vi "Wind Farm #2.vi"(8 "error in (no error)":errorcluster) -> (0 "error out":errorcluster)   [LabVIEW 2011]
doc: "This is one of 4 potential implementations for the Wind Farm Requirements. Specifically note how the wind turbine information is displayed. Also note how the main VI communicates back and forth to the wind turbine. What does that pipeline look like? Finally note the mechanism for stopping the wind turbine.\n\nAAL 9/09"
uses:
  Controls/File Type.ctl
  X Listbox Solution/X Listbox-Solution.xctl
  Shared/QDMH Poly VIs/QDMH POLY Enqueue String.vi
  Shared/QDMH Poly VIs/QDMH POLY Enqueue Cluster.vi
panel:
  in  "Wind Turbine Selection":string(xcontrol)
  in  "File Type":T1 caption="File Type (Read When Turbine is Added)"
  in  "Set Wind Speed":bool
  in  "Wind Speed":dbl=15.0
  in  "Queue Name":string
  in  "Add Wind Turbine":bool
  out "Message Display":string
  in  "Exit":bool
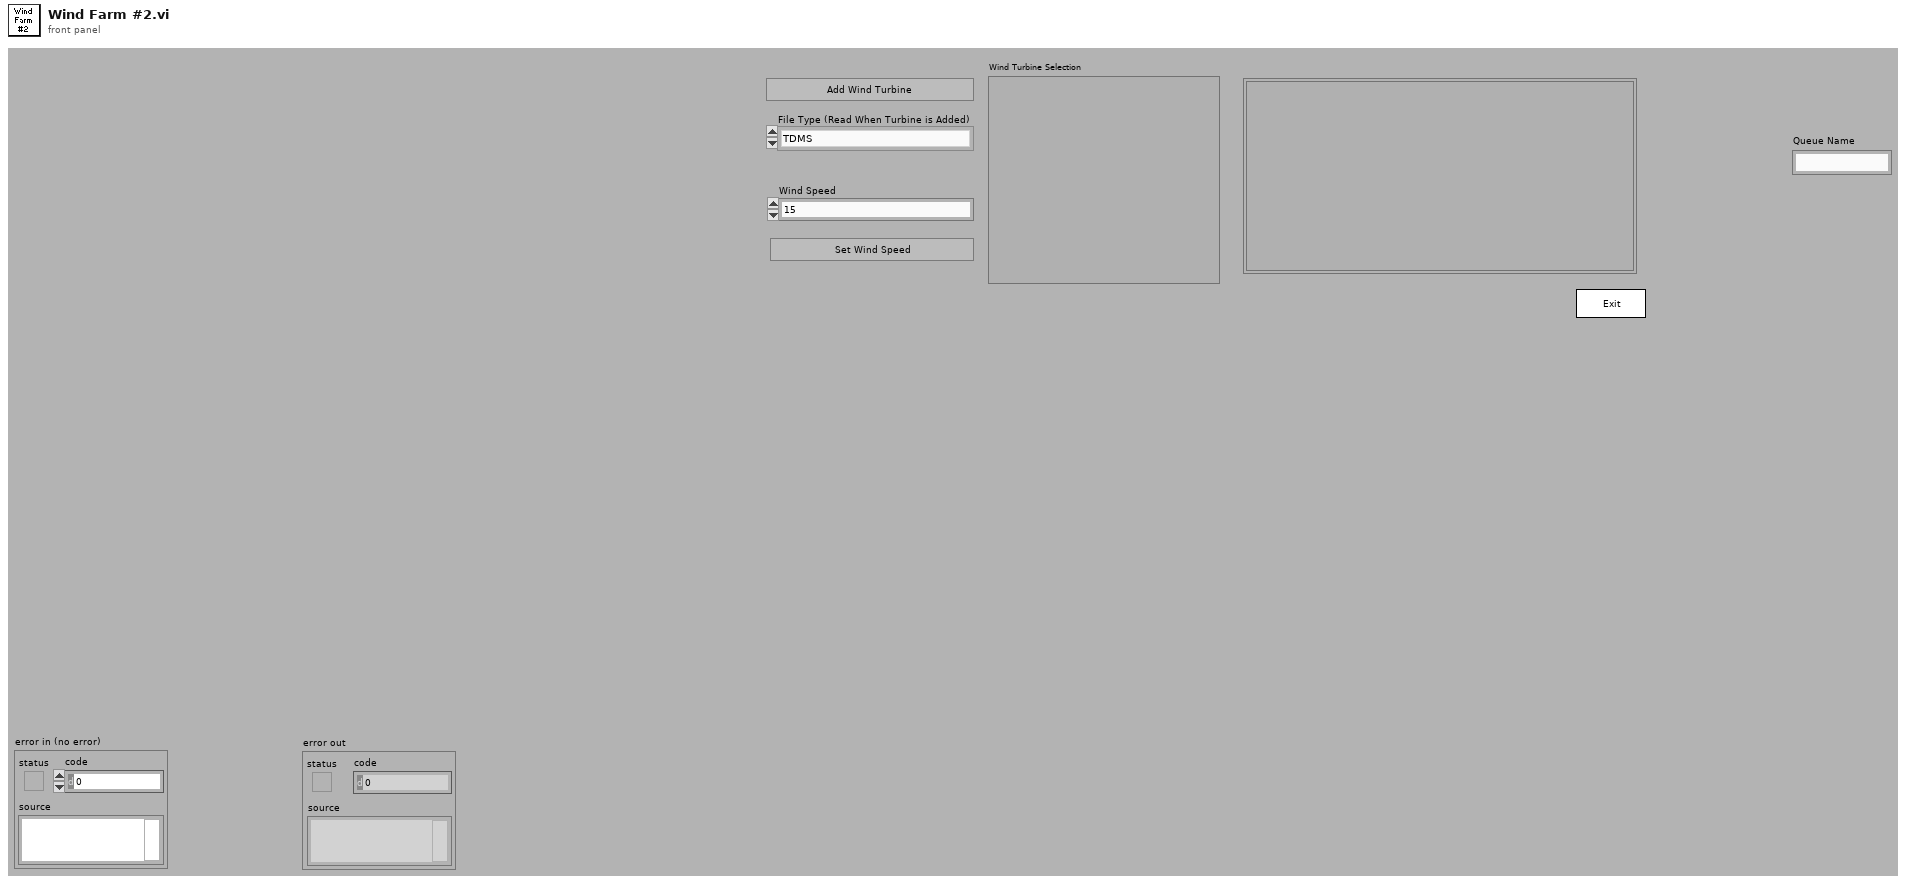
[diagram p1: front panel]
types:
  T1 = typedef "File Type.ctl" = enum16{"TDMS", "TXT"}
  T2 = cluster{"Operator Name":string, "Current VI's  Path":path, "Main Directory":path, "Y Data":dbl[], "Ini Path":path, "Model":string, "VITs Directory":path, "VIT References":refnum<vi>[], "VIT Current":refnum<vi>, "Wind Speed":dbl, "Selected Turbine":string, "Names":string[]}
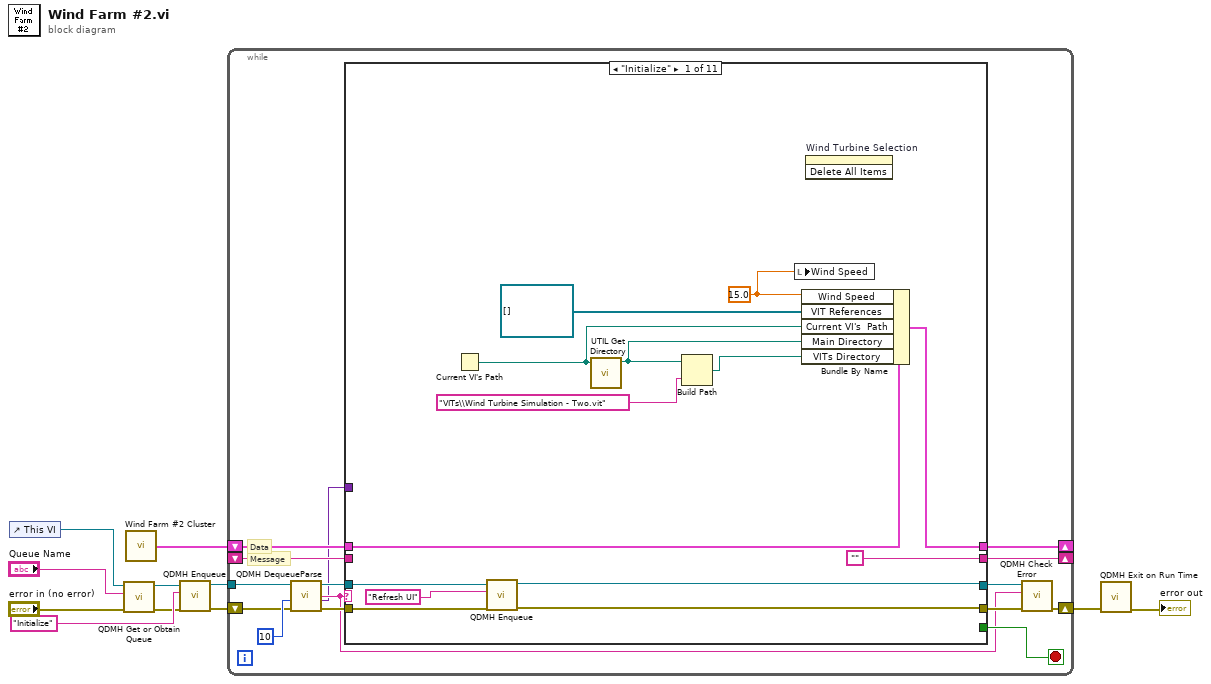
[diagram p0: block diagram]
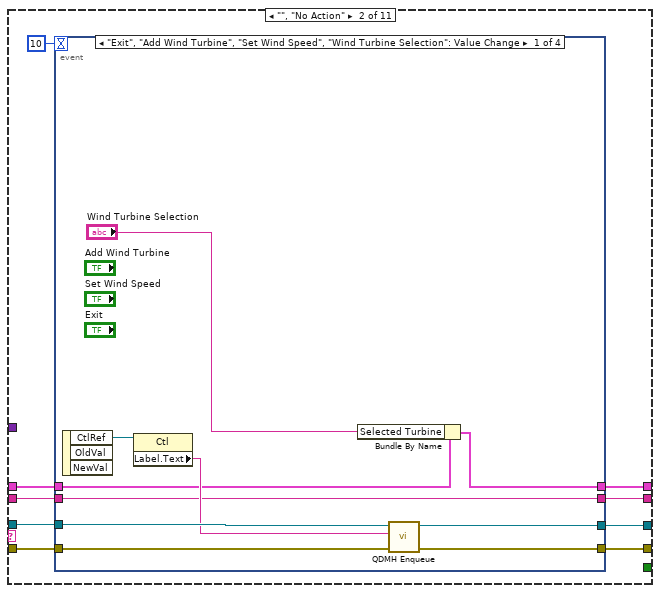
[diagram p2: hidden frame]
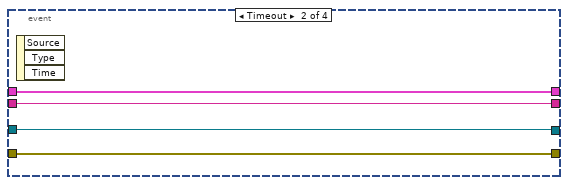
[diagram p3: hidden frame]
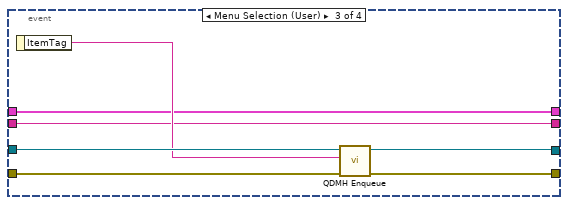
[diagram p4: hidden frame]
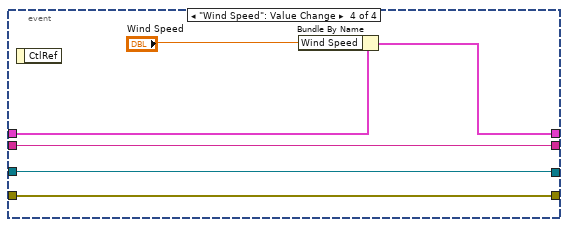
[diagram p5: hidden frame]
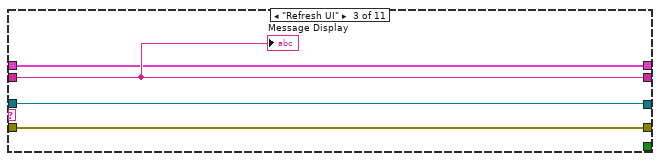
[diagram p6: hidden frame]
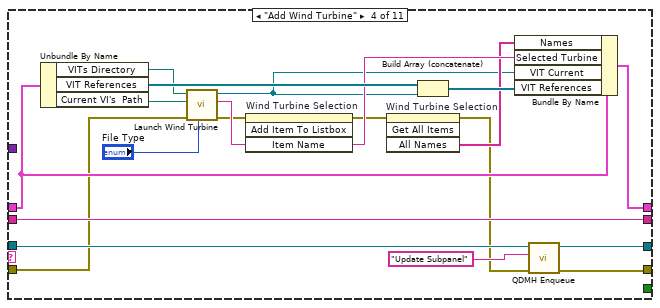
[diagram p7: hidden frame]
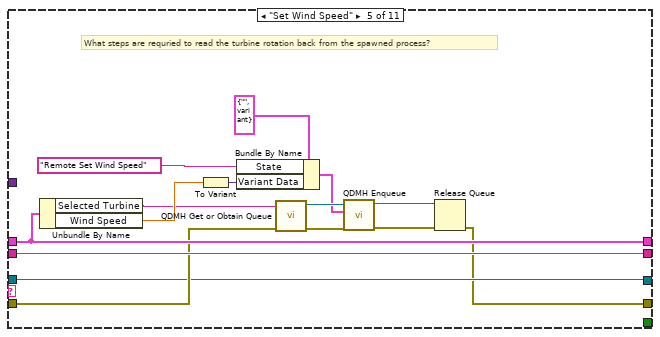
[diagram p8: hidden frame]
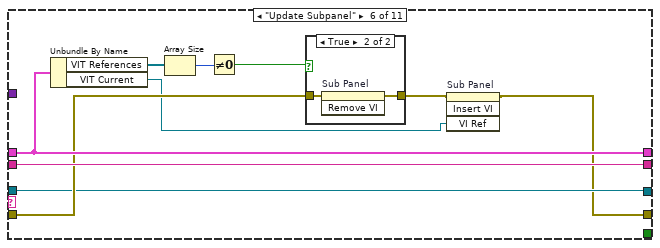
[diagram p9: hidden frame]
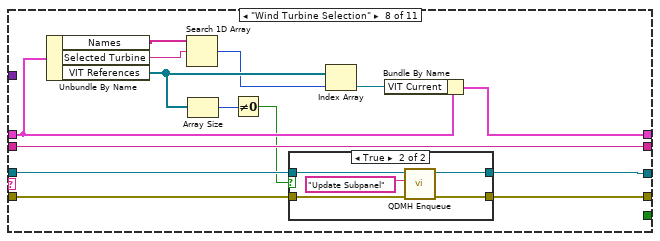
[diagram p12: hidden frame]
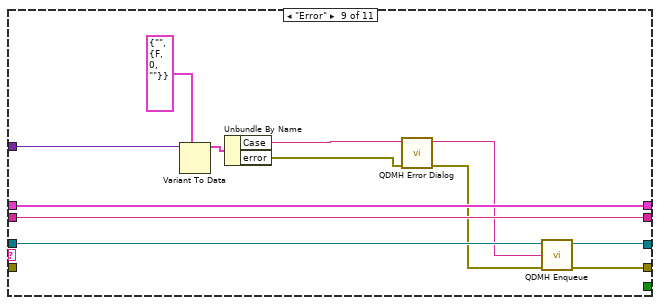
[diagram p14: hidden frame]
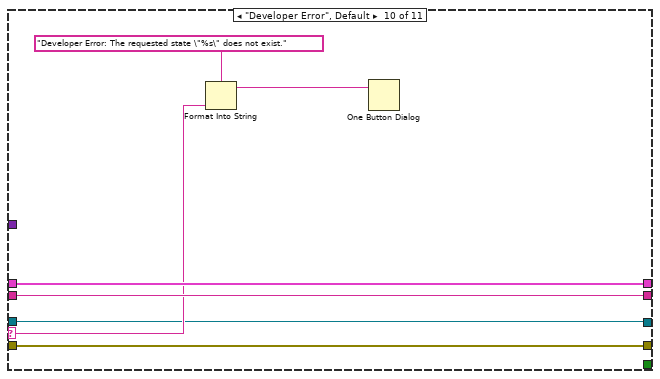
[diagram p15: hidden frame]
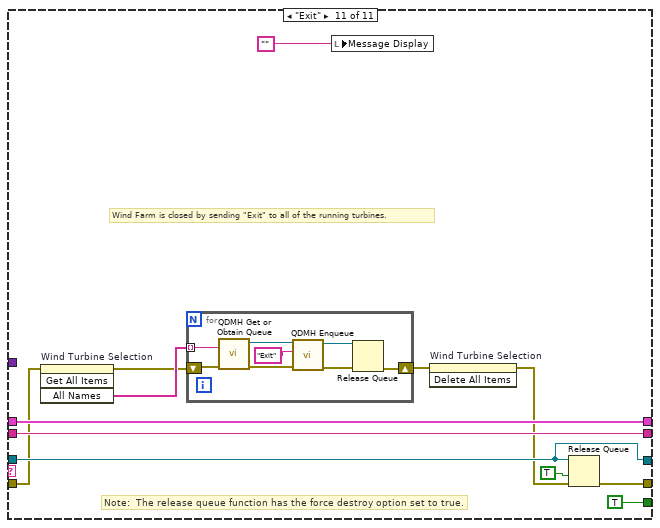
[diagram p16: hidden frame]
diagram:
  n1 = control-ref of="This VI"() -> (w1:refnum<vi>)
  n2 = call "QDMH Get or Obtain Queue.vi"("error in (no error)"="error in (no error)", "Queue Name"="Queue Name", "VI Refnum"=w1) -> ("error out"=w7:errorcluster, "queue out"=w10:refnum<queue>)  [unwired: 7 out]
  n3 = call "Wind Farm #2 Cluster.vi"() -> ("Cluster"=w3:T2)
  n4 = call-poly "QDMH Enqueue.vi"("error in (no error)"=w7, "State"="Initialize" ("element"), "queue"=w10) -> ("error out"=w8:errorcluster, "queue out"=w11:refnum<queue>)  [unwired: 7 out]
  n5 = while {
    tunnel: w11 -> [w21]
    shift-left: w3 -> [w22]
    shift-right: [w23] -> _
    shift-left: _ -> [w24]
    shift-right: [w25] -> _
    shift-right: [w15] -> w5
    shift-left: w8 -> [w17]
    stop <- w26 stop-if-true
    # "Data"
    # "Message"
    n6 = call "QDMH DequeueParse.vi"("error in (no error)"=w17, "Timeout"=10 ("ms timeout (-1)"), "queue"=w21) -> ("error out"=w18:errorcluster, "Variant Data"=w12:variant, "State"=w13:string, "queue out"=w19:refnum<queue>)  [unwired: 5 out]
    n7 = case shown="\"Initialize\"" w13 {
      selector: w13 -> [_ _ _ _ _ _ _ _ _ w168 _]
      tunnel: w19 -> [w37 w49 w77 w93 w102 w118 w128 w144 w162 w165 w180]
      tunnel: [_ _ _ _ _ _ _ _ _ _ TRUE] -> w26
      tunnel: ["" w42 w79 w99 w114 w124 w131 w145 w164 w171 w182] -> w25
      tunnel: w24 -> [_ w43 w79 w99 w114 w124 w131 w145 w164 w171 w182]
      tunnel: [w39 w44 w78 w96 w113 w123 w130 w139 w163 w170 w177] -> w23
      tunnel: w22 -> [w40 w45 w78 w97 w113 w123 w130 w140 w163 w170 w177]
      tunnel: w18 -> [w36 w48 w80 w87 w103 w119 w129 w143 _ w167 w175]
      tunnel: [w35 w47 w80 w94 w101 w117 w129 w142 w161 w167 w179] -> w16
      tunnel: [w29 w41 w77 w92 w102 w118 w128 w141 w160 w165 w180] -> w14
      tunnel: w12 -> [_ _ _ _ _ _ _ _ w155 _ _]
      frame "Initialize" {
        w28 = 15.0 ("1 Wind Speed")
        n8 = Current VI's Path() -> (path=w33:path)
        n9 = call-poly "QDMH Enqueue.vi"("error in (no error)"=w36, "State"="Refresh UI" ("element"), "queue"=w37) -> ("error out"=w35:errorcluster, "queue out"=w29:refnum<queue>)  [unwired: 7 out]
        n10 = call "UTIL Get Directory.vi"("Path In"=w33) -> ("Directory Out"=w32:path)  [unwired: 1 in, 9 out]
        n11 = Build Path(base path=w32, name or relative path="VITs\\Wind Turbine Simulation - Two.vit") -> (appended path=w31:path)
        n12 = local write "Wind Speed"(w28) -> ()
        n13 = Bundle By Name(cluster=w40, "Wind Speed"=w28, "VIT References"=refnum<vi>[] [], "Current VI's  Path"=w33, "Main Directory"=w32, "VITs Directory"=w31) -> (w39:T2)
        n14 = invoke on="Wind Turbine Selection" class="X Listbox-Solution (strict)" method="Delete All Items"() -> ()  [unwired: 3 in, 3 out]
      }
      frame "", "No Action" {
        n15 = event shown="[0] \"Exit\", \"Add Wind Turbine\", \"Set Wind Speed\", \"Wind Turbine Selection\": Value Change" {
          selector: _ -> [_ _ _ _]
          dyn-events: _ -> [_ _ _ _]
          timeout: 10 -> [_ _ _ _]
          tunnel: w49 -> [w58 w61 w70 w73]
          tunnel: [w57 w60 w68 w72] -> w47
          tunnel: w48 -> [w56 w60 w69 w72]
          tunnel: w45 -> [w52 w63 w66 w75]
          tunnel: [w51 w63 w66 w74] -> w44
          tunnel: w43 -> [w54 w62 w65 w76]
          tunnel: [w54 w62 w65 w76] -> w42
          tunnel: [w53 w61 w64 w73] -> w41
          event "Exit", "Add Wind Turbine", "Set Wind Speed", "Wind Turbine Selection": Value Change {
            n16 = event-data() -> ("CtlRef"=w59:refnum<vi>)  [unwired: 3 out]
            n17 = property class="Ctl"(reference=w59) -> ("Label.Text"=w55:string)  [unwired: 1 in, 2 out]
            n18 = Bundle By Name(cluster=w52, "Selected Turbine"="Wind Turbine Selection") -> (w51:T2)
            n19 = call-poly "QDMH Enqueue.vi"("error in (no error)"=w56, "State"=w55, "queue"=w58) -> ("error out"=w57:errorcluster, "queue out"=w53:refnum<queue>)  [unwired: 7 out]
          }
          event Timeout {
            n20 = event-data() -> ()  [unwired: 4 out]
          }
          event Menu Selection (User) {
            n21 = event-data() -> ("ItemTag"=w67:string)  [unwired: 1 out]
            n22 = call-poly "QDMH Enqueue.vi"("error in (no error)"=w69, "State"=w67, "queue"=w70) -> ("error out"=w68:errorcluster, "queue out"=w64:refnum<queue>)  [unwired: 7 out]
          }
          event "Wind Speed": Value Change {
            n23 = event-data() -> ()  [unwired: 2 out]
            n24 = Bundle By Name(cluster=w75, "Wind Speed"="Wind Speed") -> (w74:T2)
          }
        }
      }
      frame "Refresh UI" {
        "Message Display" <- w79
      }
      frame "Add Wind Turbine" {
        n25 = Unbundle By Name(w97) -> ("VITs Directory"=w90:path, "VIT References"=w91:refnum<vi>[], "Current VI's  Path"=w89:path)
        n26 = call "Launch Wind Turbine.vi"("File Type"="File Type", "error in"=w87, "Calling VI Path"=w89, "VIT Path"=w90) -> ("error out"=w83:errorcluster, "Name"=w86:string, "vi reference"=w82:refnum<vi>)  [unwired: 5 in]
        n27 = invoke on="Wind Turbine Selection" class="X Listbox-Solution (strict)" method="Add Item To Listbox"(error in=w83, "Item Name"=w86) -> (error out=w85:errorcluster)  [unwired: 2 in, 3 out]
        n28 = invoke on="Wind Turbine Selection" class="X Listbox-Solution (strict)" method="Get All Items"(error in=w85) -> (error out=w81:errorcluster, "All Names"=w84:string[])  [unwired: 3 in, 2 out]
        n29 = Build Array (concatenate)(w91, w82) -> (w98:refnum<vi>[])
        n30 = Bundle By Name(cluster=w97, "Names"=w84, "Selected Turbine"=w86, "VIT Current"=w82, "VIT References"=w98) -> (w96:T2)
        n31 = call-poly "QDMH Enqueue.vi"("error in (no error)"=w81, "State"="Update Subpanel" ("element"), "queue"=w93) -> ("error out"=w94:errorcluster, "queue out"=w92:refnum<queue>)  [unwired: 7 out]
      }
      frame "Set Wind Speed" {
        # "What steps are requried to read the turbine rotation back from the spawned process?"
        n32 = Unbundle By Name(w113) -> ("Selected Turbine"=w100:string, "Wind Speed"=w110:dbl)
        n33 = To Variant(anything=w110) -> (Variant=w109:variant)
        n34 = Bundle By Name(cluster=cluster{"State":string, "Variant Data":variant} {"State"="", "Variant Data"=variant} ("QDSM Element"), "State"="Remote Set Wind Speed", "Variant Data"=w109) -> (w106:cluster{"State":string, "Variant Data":variant})
        n35 = call "QDMH Get or Obtain Queue.vi"("error in (no error)"=w103, "Queue Name"=w100) -> ("error out"=w107:errorcluster, "queue out"=w108:refnum<queue>)  [unwired: 1 in, 7 out]
        n36 = call-poly "QDMH Enqueue.vi"("error in (no error)"=w107, "QDSM Element"=w106, "queue"=w108) -> ("error out"=w104:errorcluster, "queue out"=w105:refnum<queue>)  [unwired: 7 out]
        n37 = Release Queue(queue=w105, error in (no error)=w104) -> (error out=w101:errorcluster)  [unwired: 3 out]
      }
      frame "Update Subpanel" {
        n38 = Unbundle By Name(w123) -> ("VIT References"=w122:refnum<vi>[], "VIT Current"=w115:refnum<vi>)
        n39 = Array Size(array=w122) -> (size(s)=w121:i32)
        n40 = Not Equal To 0?(x=w121) -> (x != 0?=w120:bool)
        n41 = case shown="True" w120 {
          tunnel: w119 -> [w125 w127]
          tunnel: [w125 w126] -> w116
          frame False {
          }
          frame True {
            n42 = invoke on="Sub Panel" class="SubPnl" method="Remove VI"(error in=w127) -> (error out=w126:errorcluster)  [unwired: 2 in, 2 out]
          }
        }
        n43 = invoke on="Sub Panel" class="SubPnl" method="Insert VI"(error in=w116, "VI Ref"=w115) -> (error out=w117:errorcluster)  [unwired: 2 in, 3 out]
      }
      frame "<add states as needed>" {
        # "Duplicate this state for any additional states that you add."
      }
      frame "Wind Turbine Selection" {
        n44 = Unbundle By Name(w140) -> ("Names"=w134:string[], "Selected Turbine"=w133:string, "VIT References"=w137:refnum<vi>[])
        n45 = Search 1D Array(1D array=w134, element=w133) -> (index of element=w135:i32)  [unwired: 1 in]
        n46 = Array Size(array=w137) -> (size(s)=w136:i32)
        n47 = Not Equal To 0?(x=w136) -> (x != 0?=w132:bool)
        n48 = case shown="True" w132 {
          tunnel: w144 -> [w147 w152]
          tunnel: w143 -> [w146 w151]
          tunnel: [w146 w150] -> w142
          tunnel: [w147 w149] -> w141
          frame False {
          }
          frame True {
            n49 = call-poly "QDMH Enqueue.vi"("error in (no error)"=w151, "State"="Update Subpanel", "queue"=w152) -> ("error out"=w150:errorcluster, "queue out"=w149:refnum<queue>)  [unwired: 7 out]
          }
        }
        n50 = Index Array(array=w137, index=w135) -> (element=w138:refnum<vi>)
        n51 = Bundle By Name(cluster=w140, "VIT Current"=w138) -> (w139:T2)
      }
      frame "Error" {
        n52 = Variant To Data(type=cluster{"Case":string, "error":errorcluster} {"Case"="", "error"={"status"=FALSE, "code"=0, "source"=""}} ("QDSM Element"), Variant=w155) -> (data=w158:cluster{"Case":string, "error":errorcluster})  [unwired: 1 in, 1 out]
        n53 = Unbundle By Name(w158) -> ("Case"=w157:string, "error"=w156:errorcluster)
        n54 = call "QDMH Error Dialog.vi"("error"=w156, "Case Error Occured"=w157) -> ("error out (no error)"=w153:errorcluster, "Case to Execute"=w154:string)  [unwired: 8 out]
        n55 = call-poly "QDMH Enqueue.vi"("error in (no error)"=w153, "State"=w154, "queue"=w162) -> ("error out"=w161:errorcluster, "queue out"=w160:refnum<queue>)  [unwired: 7 out]
      }
      frame "Developer Error", Default {
        n56 = Format Into String(format string="Developer Error: The requested state \"%s\" does not exist." ("message"), w168) -> (resulting string=w166:string)  [unwired: 2 in, 1 out]
        n57 = One Button Dialog(message=w166) -> ()  [unwired: 2 out]
      }
      frame "Exit" {
        # "Wind Farm is closed by sending \"Exit\" to all of the running turbines."
        # "Note:  The release queue function has the force destroy option set to true."
        n58 = invoke on="Wind Turbine Selection" class="X Listbox-Solution (strict)" method="Get All Items"(error in=w175) -> (error out=w174:errorcluster, "All Names"=w176:string[])  [unwired: 3 in, 2 out]
        n59 = for {
          tunnel: w176 -> [w191] mode=indexing
          shift-right: [w184] -> w173
          shift-left: w174 -> [w186]
          n60 = call "QDMH Get or Obtain Queue.vi"("error in (no error)"=w186, "Queue Name"=w191) -> ("error out"=w185:errorcluster, "queue out"=w190:refnum<queue>)  [unwired: 1 in, 7 out]
          n61 = call-poly "QDMH Enqueue.vi"("error in (no error)"=w185, "State"="Exit", "queue"=w190) -> ("error out"=w187:errorcluster, "queue out"=w188:refnum<queue>)  [unwired: 7 out]
          n62 = Release Queue(queue=w188, error in (no error)=w187) -> (error out=w184:errorcluster)  [unwired: 1 in, 2 out]
        }
        n63 = local write "Message Display"("") -> ()
        n64 = invoke on="Wind Turbine Selection" class="X Listbox-Solution (strict)" method="Delete All Items"(error in=w173) -> (error out=w172:errorcluster)  [unwired: 2 in, 2 out]
        n65 = Release Queue(queue=w180, force destroy? (F)=TRUE, error in (no error)=w172) -> (error out=w179:errorcluster)  [unwired: 2 out]
      }
    }
    n66 = call "QDMH Check Error.vi"("error in (no error)"=w16, "Case"=w13, "queue"=w14) -> ("error out"=w15:errorcluster)  [unwired: 1 in, 7 out]
  }
  n67 = call "QDMH Exit on Run Time.vi"("error in (no error)"=w5) -> ("error out"=→"error out":errorcluster)  [unwired: 10 out]
